vi "Manipulator Controller.vi"   [LabVIEW 2018]
uses:
  <vilib>/Rock Robotics/WPI/Joystick/WPI_JoystickDeviceEnum.ctl
  Manipulator Controller Global.vi
types:
  T1 = typedef "WPI_JoystickDeviceEnum.ctl" = enum16{"USB 0", "USB 1", "USB 2", "USB 3", "USB 4", "USB 5"}
  T2 = typedef "WPI_JoystickDevRef.ctl" = cluster{"Device":T1}
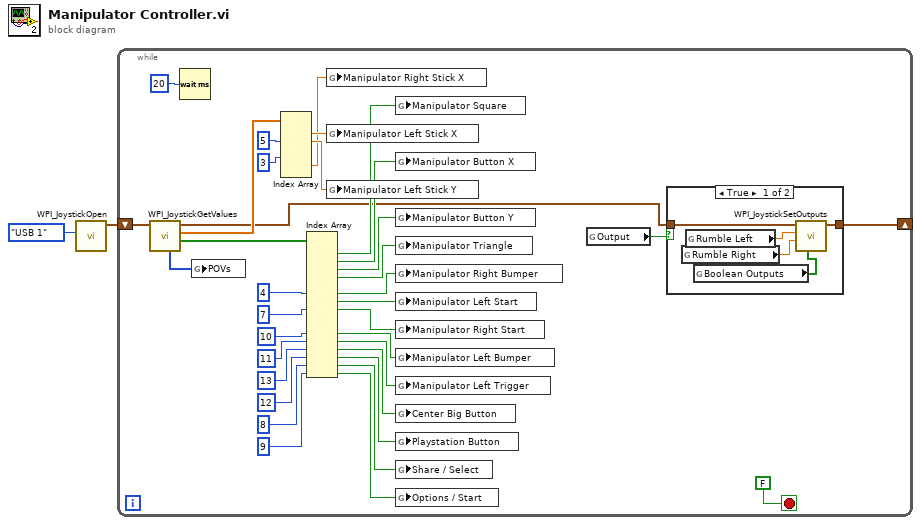
[diagram p0: block diagram]
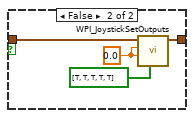
[diagram p2: hidden frame]
diagram:
  n1 = call <vilib>:"WPI_JoystickOpen.vi"("JoystickDevice"=WPI_JoystickDeviceEnum."USB 1") -> ("JoystickDevRef"=w1:T2)  [unwired: 10 in]
  n2 = while {
    shift-right: [w3] -> _
    shift-left: w1 -> [w37]
    stop <- FALSE stop-if-true
    n3 = call <vilib>:"WPI_JoystickGetValues.vi"("JoystickDevRef"=w37) -> ("Buttons"=w35:bool[], "Axes"=w36:dbl[], "JoystickDevRef"=w5:T2, "POVs"=w19:i16[])  [unwired: 6 in, 1 out]
    n4 = Wait (ms)(milliseconds to wait=u32 20) -> ()  [unwired: 1 out]
    n5 = global write "Manipulator Controller Global.vi" "POVs"(w19) -> ()
    n6 = Index Array(array=w36, index #2=5 ("index"), index #4=3 ("index")) -> (element #1=w34:dbl, element #2=w33:dbl, element #5=w32:dbl)  [unwired: 4 in, 3 out]
    n7 = Index Array(array=w35, index #6=4 ("index"), index #8=7 ("index"), index #11=10 ("index"), index #12=11 ("index"), index #13=13 ("index"), index #14=12 ("index"), index #15=8 ("index"), index #16=9 ("index")) -> (element #1=w31:bool, element #2=w30:bool, element #3=w29:bool, element #4=w18:bool, element #6=w28:bool, element #7=w27:bool, element #8=w26:bool, element #11=w16:bool, element #12=w14:bool, element #13=w12:bool, element #14=w10:bool, element #15=w7:bool, element #16=w6:bool)  [unwired: 8 in, 3 out]
    n8 = global write "Manipulator Controller Global.vi" "Manipulator Right Stick X"(w32) -> ()
    n9 = global write "Manipulator Controller Global.vi" "Manipulator Left Stick X"(w34) -> ()
    n10 = global write "Manipulator Controller Global.vi" "Manipulator Left Stick Y"(w33) -> ()
    n11 = global write "Manipulator Controller Global.vi" "Manipulator Square"(w31) -> ()
    n12 = global write "Manipulator Controller Global.vi" "Manipulator Button X"(w30) -> ()
    n13 = global write "Manipulator Controller Global.vi" "Manipulator Button Y"(w29) -> ()
    n14 = global write "Manipulator Controller Global.vi" "Manipulator Triangle"(w18) -> ()
    n15 = global write "Manipulator Controller Global.vi" "Manipulator Right Bumper"(w28) -> ()
    n16 = global write "Manipulator Controller Global.vi" "Manipulator Left Start"(w27) -> ()
    n17 = global write "Manipulator Controller Global.vi" "Manipulator Right Start"(w26) -> ()
    n18 = global write "Manipulator Controller Global.vi" "Manipulator Left Bumper"(w16) -> ()
    n19 = global write "Manipulator Controller Global.vi" "Manipulator Left Trigger"(w14) -> ()
    n20 = global write "Manipulator Controller Global.vi" "Center Big Button"(w12) -> ()
    n21 = global write "Manipulator Controller Global.vi" "Playstation Button"(w10) -> ()
    n22 = global write "Manipulator Controller Global.vi" "Share / Select"(w7) -> ()
    n23 = global write "Manipulator Controller Global.vi" "Options / Start"(w6) -> ()
    n24 = global read "Manipulator Controller Global.vi" "Output"() -> (w4:bool)
    n25 = case shown="True" w4 {
      tunnel: [w42 w46] -> w3
      tunnel: w5 -> [w41 w45]
      frame True {
        n26 = global read "Manipulator Controller Global.vi" "Rumble Right"() -> (w39:dbl)
        n27 = global read "Manipulator Controller Global.vi" "Rumble Left"() -> (w38:dbl)
        n28 = global read "Manipulator Controller Global.vi" "Boolean Outputs"() -> (w40:bool[])
        n29 = call <vilib>:"WPI_JoystickSetOutputs.vi"("Outputs"=w40, "Right Rumble"=w39, "Left Rumble"=w38, "JoystickDevRef"=w41) -> ("JoystickDevRef"=w42:T2)  [unwired: 6 in, 1 out]
      }
      frame False {
        w44 = sgl 0.0 ("Left Rumble")
        n30 = call <vilib>:"WPI_JoystickSetOutputs.vi"("Outputs"=bool[] [TRUE, TRUE, TRUE, TRUE, TRUE], "Right Rumble"=w44, "Left Rumble"=w44, "JoystickDevRef"=w45) -> ("JoystickDevRef"=w46:T2)  [unwired: 6 in, 1 out]
      }
    }
  }
